vi "TCP Data Stream PC.vi"(0 "RT IP Address":string, 5 "Error IN":errorcluster, 6 "Mode":T1) -> (14 "Data OUT":dbl[][](array[numeric]), 15 "New Data?":bool, 16 "Connected?":bool, 19 "Error OUT":errorcluster)   [LabVIEW 2019]
uses:
  Type Defs/TCP Data Stream Mode (PC).ctl
  Type Defs/TCP Data Stream Mode.ctl
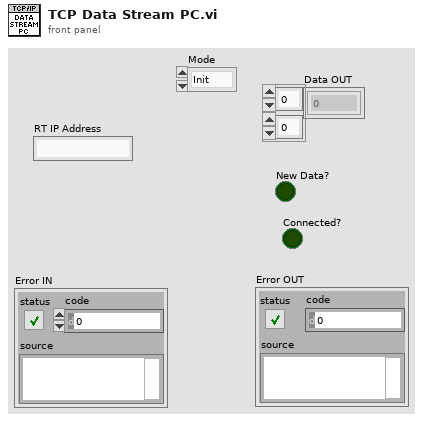
[diagram p1: front panel]
types:
  T1 = typedef "TCP Data Stream Mode (PC).ctl" = enum16{"Init", "Read Data", "Close"}
  T2 = typedef "TCP Data Stream Mode.ctl" = enum16{"Init RT", "Init PC", "Connect RT", "Connect PC", "Write Data", "Read Data", "Close"}
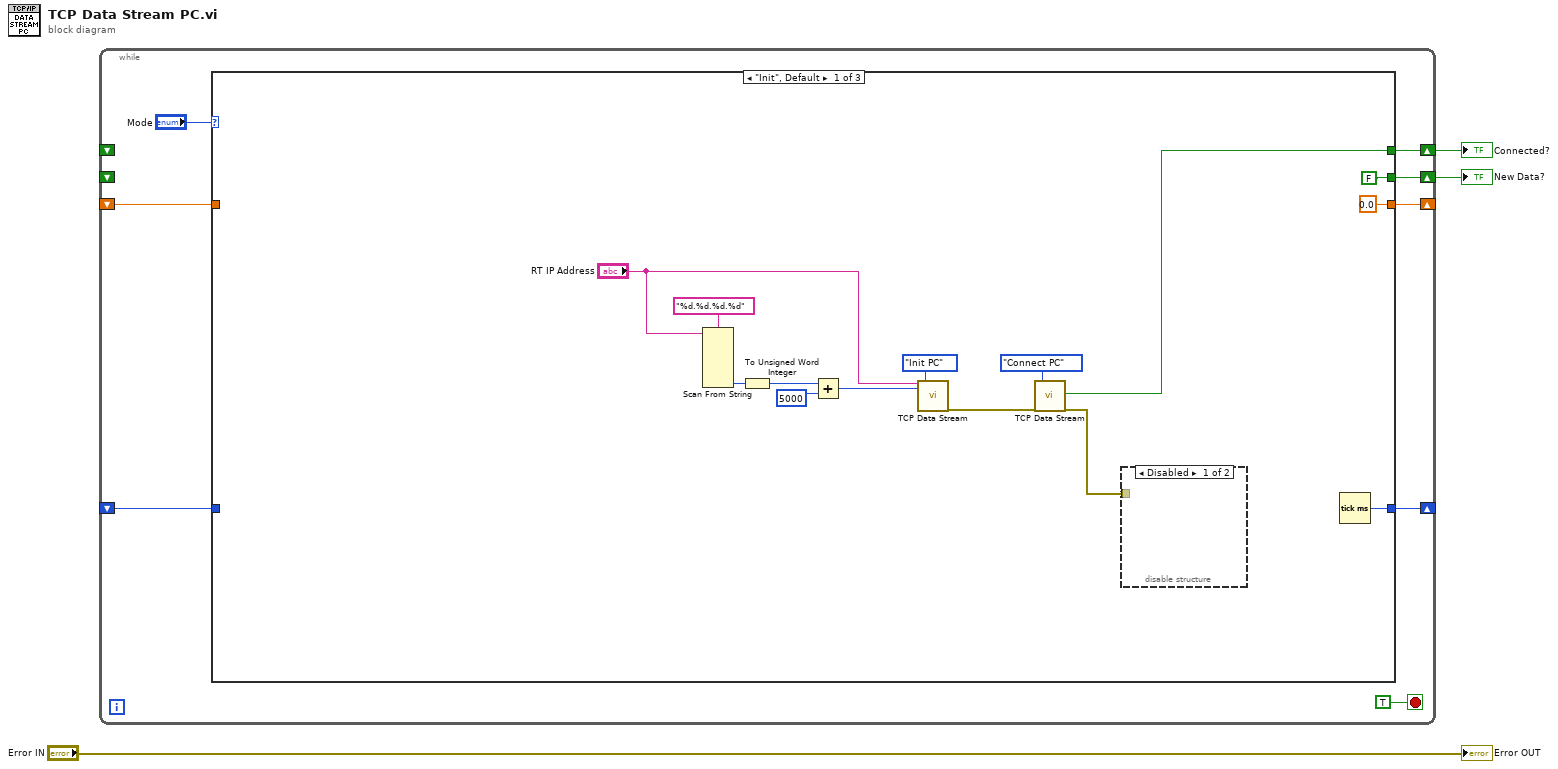
[diagram p0: block diagram]
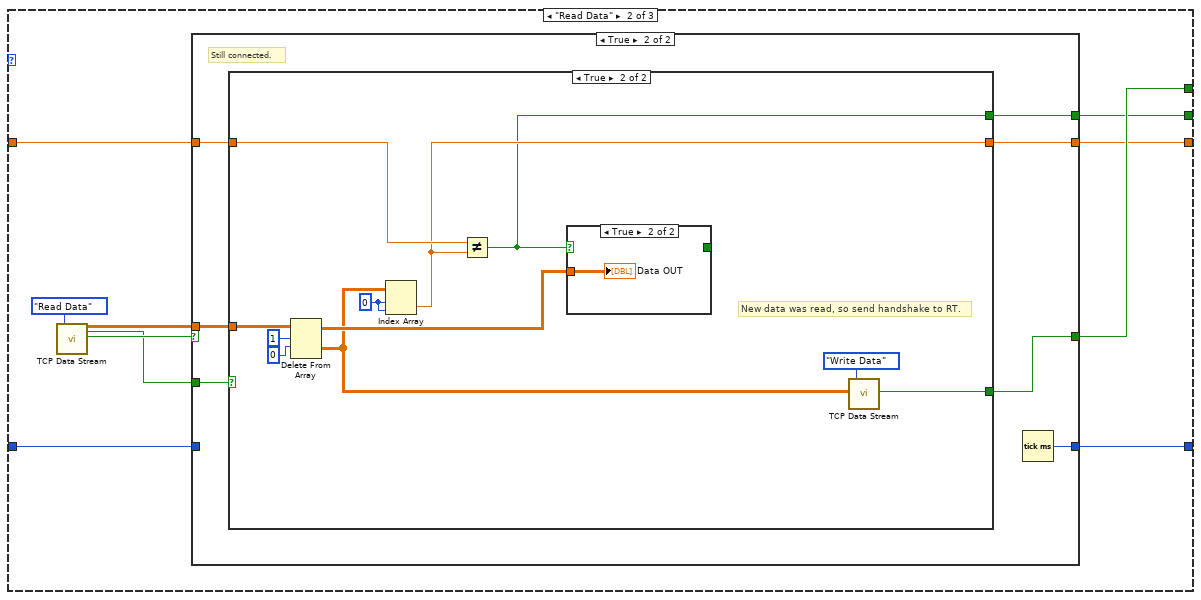
[diagram p3: hidden frame]
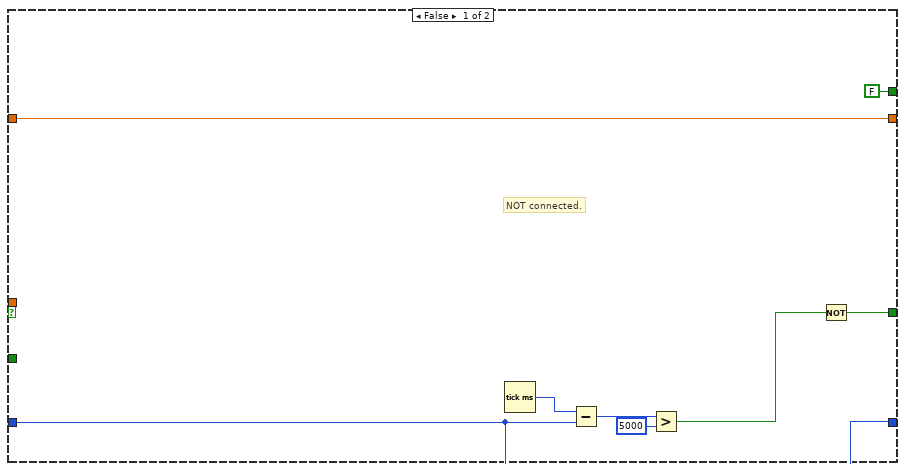
[diagram p4: hidden frame]
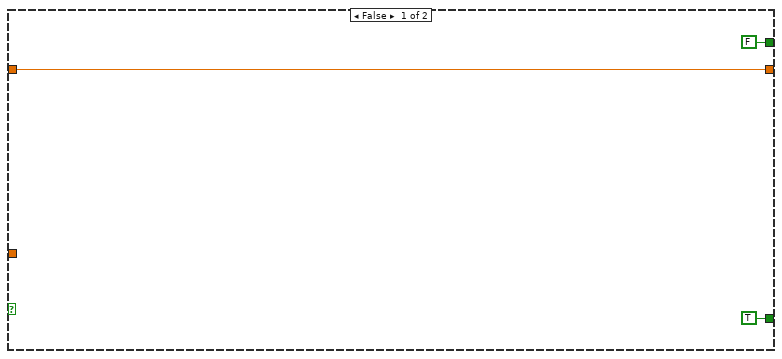
[diagram p5: hidden frame]
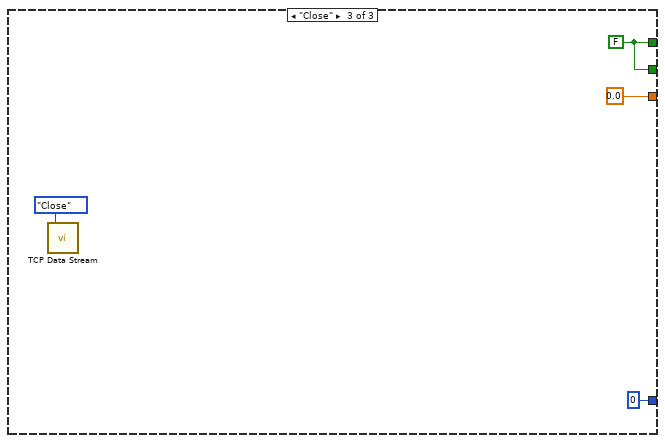
[diagram p7: hidden frame]
diagram:
  n1 = while {
    shift-right: [w9] -> w2
    shift-left: _ -> [_]
    shift-right: [w8] -> w1
    shift-left: _ -> [_]
    shift-right: [w7] -> _
    shift-left: _ -> [w6]
    shift-right: [w5] -> _
    shift-left: _ -> [w4]
    stop <- TRUE stop-if-true
    n2 = case shown="\"Init\", Default" "Mode" {
      tunnel: [w14 w33 w70] -> w9
      tunnel: [FALSE ("Connected?") w26 w70] -> w8
      tunnel: [w15 w31 u32 0 ("millisecond timer value")] -> w7
      tunnel: w6 -> [_ w32 _]
      tunnel: [0.0 w27 0.0] -> w5
      tunnel: w4 -> [_ w28 _]
      frame "Init", Default {
        n3 = Scan From String(format string="%d.%d.%d.%d", input string="RT IP Address") -> (output 4=w24:i32)  [unwired: 9 in, 3 out]
        n4 = To Unsigned Word Integer(number=w24) -> (unsigned 16bit integer=w22:u16)
        n5 = Add(x=w22, y=u16 5000 ("Port")) -> (x+y=w16:u16)
        n6 = call "TCP Data Stream.vi"("Address"="RT IP Address", "Port"=w16, "Mode"=TCP_Data_Stream_Mode."Init PC") -> ("Error OUT"=w17:errorcluster)  [unwired: 12 in, 4 out]
        n7 = call "TCP Data Stream.vi"("Error IN"=w17, "Mode"=TCP_Data_Stream_Mode."Connect PC") -> ("Connected?"=w14:bool, "Error OUT"=w12:errorcluster)  [unwired: 13 in, 3 out]
        n8 = disable-structure shown="Disabled" {
          disable-tunnel: w12 -> [_ _]
          frame Disabled {
          }
          frame Enabled {
          }
        }
        n9 = Tick Count (ms)() -> (millisecond timer value=w15:u32)
      }
      frame "Read Data" {
        n10 = call "TCP Data Stream.vi"("Mode"=TCP_Data_Stream_Mode."Read Data") -> ("Data OUT"=w29:dbl[][], "New Data?"=w30:bool, "Connected?"=w34:bool)  [unwired: 14 in, 2 out]
        n11 = case shown="True" w34 {
          tunnel: w30 -> [_ w50]
          tunnel: [w40 w49] -> w33
          tunnel: w32 -> [w38 _]
          tunnel: [w38 w48] -> w31
          tunnel: w29 -> [_ w47]
          tunnel: w28 -> [w37 w46]
          tunnel: [w37 w45] -> w27
          tunnel: [FALSE w44] -> w26
          frame False {
            # "NOT connected."
            n12 = Tick Count (ms)() -> (millisecond timer value=w39:u32)
            n13 = Subtract(x=w39, y=w38) -> (x-y=w43:u32)
            n14 = Greater?(x=w43, y=u32 5000) -> (0:w41:bool)
            n15 = Not(x=w41) -> (.not. x?=w40:bool)
          }
          frame True {
            # "Still connected."
            n16 = case shown="True" w50 {
              tunnel: [TRUE ("Connected?") w64] -> w49
              tunnel: w47 -> [_ w60]
              tunnel: w46 -> [w52 w59]
              tunnel: [w52 w58] -> w45
              tunnel: [FALSE w54] -> w44
              frame False {
              }
              frame True {
                w55 = 0 ("index (row)")
                # "New data was read, so send handshake to RT."
                n17 = Delete From Array(array=w60, length=1, index (row)=0) -> (deleted portion=w56:dbl[][], array with subset deleted=w63:dbl[][])  [unwired: 1 in]
                n18 = Index Array(array=w56, index (row)=w55, index (col)=w55) -> (element=w58:dbl)
                n19 = Not Equal?(x=w59, y=w58) -> (x != y?=w54:bool)
                n20 = case shown="True" w54 {
                  selector: w54 -> [w65 _]
                  tunnel: w63 -> [_ w66]
                  tunnel: [w65 _] -> _
                  frame False {
                  }
                  frame True {
                    "Data OUT" <- w66
                  }
                }
                n21 = call "TCP Data Stream.vi"("Data IN"=w56, "Mode"=TCP_Data_Stream_Mode."Write Data") -> ("Connected?"=w64:bool)  [unwired: 13 in, 4 out]
              }
            }
            n22 = Tick Count (ms)() -> (millisecond timer value=w48:u32)
          }
        }
      }
      frame "Close" {
        w70 = FALSE ("Connected?")
        n23 = call "TCP Data Stream.vi"("Mode"=TCP_Data_Stream_Mode."Close") -> ()  [unwired: 14 in, 5 out]
      }
    }
  }
  "Connected?" <- w2
  "New Data?" <- w1
  "Error OUT" <- "Error IN"
